vi "Test Namer with Folder non-default folder no extension no label.vi"   [LabVIEW 2020, in "Namer.Tests.lvclass"]
uses:
  Namer.Tests.lvclass
  Source/Approval Tests/Namer with Folder/Namer with Folder.lvclass
  Source/Approval Tests/Naming Data/Naming Data.lvclass
  Source/Approval Tests/Namer with Folder/Namer with Folder.lvclass/Namer with Folder.ctl
  Source/Approval Tests/Naming Data/Naming Data.lvclass/Naming Data.ctl
  Source/Approval Tests/Naming Data/Write Test VI Name.vi
  Source/Approval Tests/Namer with Folder/Write Relative Folder Path.vi
  <vilib>/addons/_JKI Toolkits/Caraya/classes/Assert/Assert Equal Value and Type_Variant.vi
  <vilib>/addons/_JKI Toolkits/Caraya/classes/Test/Test.lvclass
  <vilib>/addons/_JKI Toolkits/Caraya/classes/Assert/Assert.lvclass
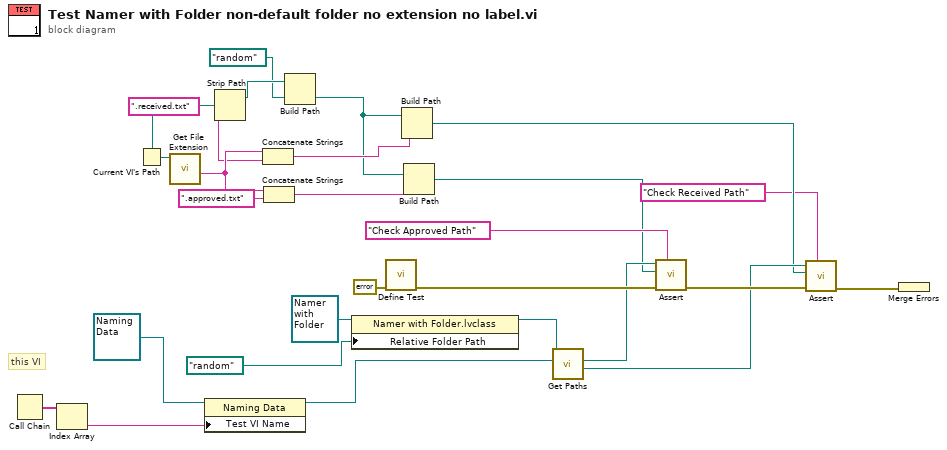
[diagram p0: block diagram]
diagram:
  # "this VI"
  n1 = Call Chain() -> (call chain=w21:string[])
  n2 = Index Array(array=w21) -> (element=w20:string)  [unwired: 1 in]
  n3 = Current VI's Path() -> (path=w14:path)
  n4 = call <vilib>:"Get File Extension.vi"("file"=w14) -> ("filename without extension"=w13:string)  [unwired: 6 in, 4 out]
  n5 = property on="Property Node" class="Naming Data"(reference=refnum<class "Naming Data.lvclass"> refnum ("Naming Data"), "Test VI Name"=w20) -> (reference out=w19:refnum<class "Naming Data.lvclass">)  [unwired: 1 in, 1 out]
  n6 = Strip Path(path=w14) -> (stripped path=w4:path)  [unwired: 1 out]
  n7 = Concatenate Strings(w13, ".received.txt" ("string")) -> (w10:string)
  n8 = Concatenate Strings(w13, ".approved.txt" ("string")) -> (w9:string)
  n9 = Build Path(base path=w4, name or relative path=path "random") -> (appended path=w5:path)
  n10 = property class="Namer with Folder.lvclass"(reference=refnum<class "Namer with Folder.lvclass"> refnum ("Approval Tests:Namer with SubFolder.lvclass"), "Relative Folder Path"=path "random") -> (reference out=w2:refnum<class "Namer with Folder.lvclass">)  [unwired: 1 in, 1 out]
  n11 = call <vilib>:"Define Test.vi"("error in (no error)"=errorcluster {"status"=FALSE, "code"=0, "source"=""}) -> ("error out"=w25:errorcluster)  [unwired: 9 in, 1 out]
  n12 = Build Path(base path=w5, name or relative path=w10) -> (appended path=w8:path)
  n13 = Build Path(base path=w5, name or relative path=w9) -> (appended path=w7:path)
  n14 = call-dynamic "Get Paths.vi"("Naming Data"=w19, "Namer with Folder in"=w2) -> ("Received Path"=w15:path, "Approved Path"=w16:path)  [unwired: 6 in, 2 out]
  n15 = call-poly <vilib>:"Assert.vi"("Label"="Check Approved Path" ("Label (VI Title)"), "error in (no error)"=w25, "Y"=w7, "X"=w16) -> ("error out"=w18:errorcluster)  [unwired: 6 in, 1 out]
  n16 = call-poly <vilib>:"Assert.vi"("Label"="Check Received Path" ("Label (VI Title)"), "error in (no error)"=w18, "Y"=w8, "X"=w15) -> ("error out"=w17:errorcluster)  [unwired: 6 in, 1 out]
  n17 = Merge Errors(w17) -> ()  [unwired: 1 out]
